vi "FiberMRI_Main.vi"() -> ()   [LabVIEW 2010]
doc: "Acquisition software for combined single-photon fluorescence and fMRI experiments."
uses:
  typedefs/acquisition_parameters_cluster.ctl
  typedefs/storage_parameters_cluster.ctl
  typedefs/experiment_mode_enum.ctl
  typedefs/stimulation_parameters.ctl
  typedefs/main_state_enum.ctl
  typedefs/control_daq_enum.ctl
  typedefs/control_display_enum.ctl
  typedefs/control_storage_enum.ctl
  typedefs/control_analysis_enum.ctl
  <vilib>/Utility/error.llb/DialogType.ctl
  typedefs/all_frontpanel_parameters.ctl
  <vilib>/ULx/Create Channel.llb/ULx Create Channel (DO-Digital Output).vi
  <vilib>/ULx/Write.llb/ULx Write (Digital Bool 1Line 1Point).vi
  globals/exit.vi
panel:
  out "Running":bool
  in  "Stimulation parameters":T1={"Physical channel"="Dev0/1stPortB/Do0", "Write chunk size"=1, "Sample rate"=1.0, "Stim onset"=0.0, "Stim frequency"=1.0, "ON time"=40.0, "OFF time"=120.0, "Repetitions"=1.0} {"Write chunk size" min=100 max=100000; "Sample rate" min=10.0 max=10000.0; "Repetitions" min=0.0 max=10.0 step=1.0; "OFF time" min=0.0 max=1000.0; "ON time" min=0.0 max=1000.0; "Stim onset" min=0.0 max=100.0; "Stim frequency" min=1.0 max=40.0 step=1.0}
  in  "Reset":bool
  in  "Shutter":bool
  in  "Experiment mode":T2
  in  "Storage parameters":T3
  in  "Acquisition parameters":T4={"Physical channels"="Dev0/Ai0:1", "Shutter line"="Dev0/1stPortA/Do0", "Clock source"=0, "Triggered?"=FALSE, "Sample rate"=1000.0, "Pixels to integrate"=1, "Effective data rate"=2000.0, "Read chunk size"=0, "Samples to read"=2000, "Run mode"=enum."Continuously"} {"Pixels to integrate" min=1 step=1; "Sample rate" min=10.0 max=25000.0; "Clock source" items=["OnboardClock", "ExternalClock", "NoClock"]}
  in  "Run":bool
  in  "Quit":bool
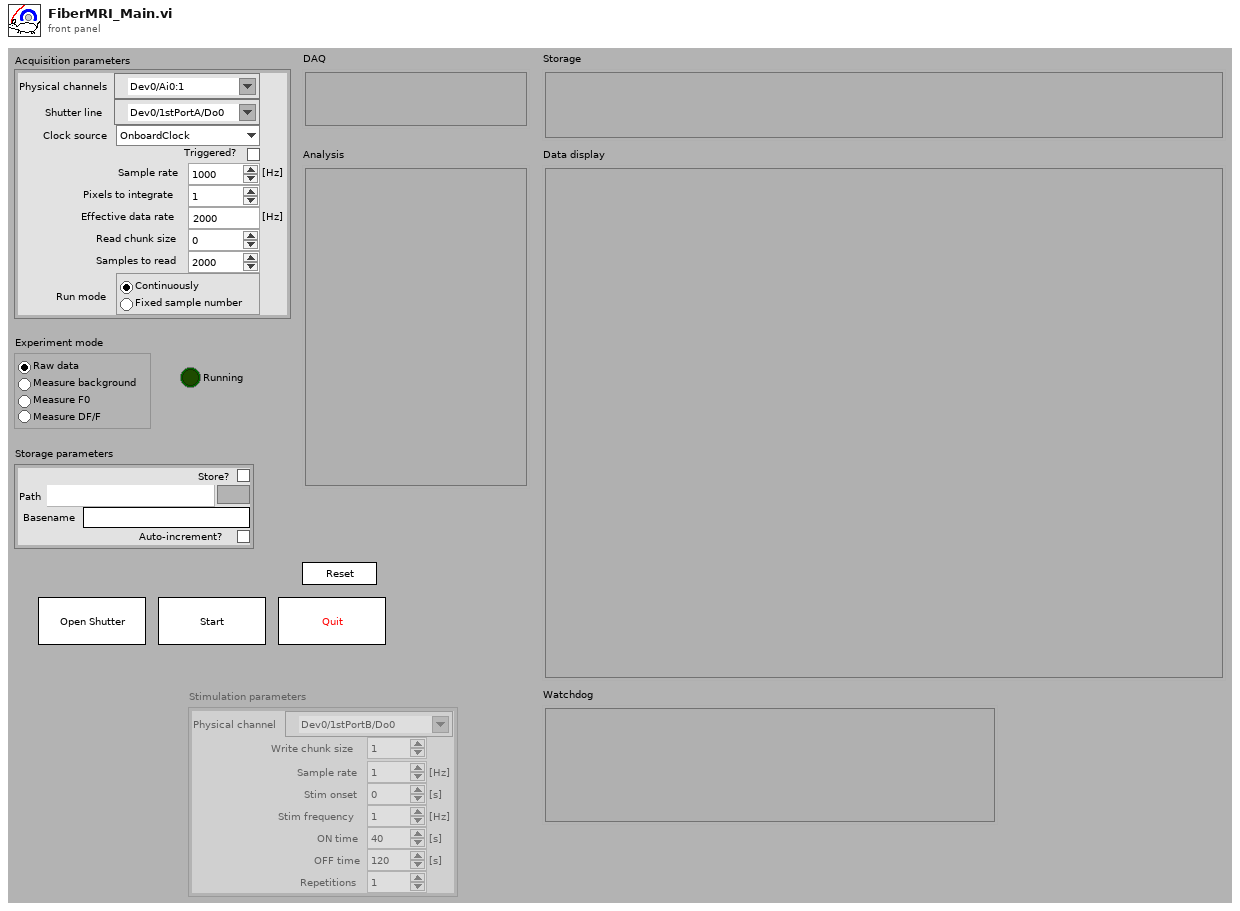
[diagram p1: front panel]
types:
  T1 = typedef "stimulation_parameters.ctl" = cluster{"Physical channel":tag, "Write chunk size":i32, "Sample rate":dbl, "Stim onset":dbl, "Stim frequency":dbl, "ON time":dbl, "OFF time":dbl, "Repetitions":dbl}
  T2 = typedef "experiment_mode_enum.ctl" = enum32{"Raw data", "Measure background", "Measure F0", "Measure DF/F"}
  T3 = typedef "storage_parameters_cluster.ctl" = cluster{"Store?":bool, "Path":path, "Basename":string, "Auto-increment?":bool}
  T4 = typedef "acquisition_parameters_cluster.ctl" = cluster{"Physical channels":refnum<k21>, "Shutter line":refnum<k21>, "Clock source":i32, "Triggered?":bool, "Sample rate":dbl, "Pixels to integrate":i32, "Effective data rate":dbl, "Read chunk size":i32, "Samples to read":i32, "Run mode":enum32{"Continuously", "Fixed sample number"}}
  T5 = typedef "all_frontpanel_parameters.ctl" = cluster{"Acquisition parameters":T4, "Experiment mode":T2, "Storage parameters":T3, "Stimulation parameters":T1}
  T6 = typedef "DialogType.ctl" = u16
  T7 = typedef "main_state_enum.ctl" = enum16{"Init", "ParamsChanged", "Start", "Stop", "SetShutter", "Reset", "Save", "Quit"}
  T8 = cluster{"Control_DAQ_Queue":refnum<queue>, "Control_Storage_Queue":refnum<queue>, "Control_Display_Queue":refnum<queue>, "Control_Analysis_Queue":refnum<queue>}
  T9 = typedef "control_analysis_enum.ctl" = enum16{"Init", "Analyze", "Reset", "Stop", "Quit"}
  T10 = cluster{"Control Analysis Enum":T9, "variant":variant}
  T11 = typedef "control_display_enum.ctl" = enum16{"Init", "Display", "Quit"}
  T12 = cluster{"Control display enum":T11, "variant":variant}
  T13 = typedef "control_storage_enum.ctl" = enum16{"Init", "Discard", "Store", "Reset", "Stop", "Quit"}
  T14 = cluster{"Control storage enum":T13, "variant":variant}
  T15 = typedef "control_daq_enum.ctl" = enum16{"Init", "GetCont", "GetNoSamples", "Stop", "Quit"}
  T16 = cluster{"Control DAQ Enum":T15, "variant":variant}
  T17 = cluster{"Acquisition parameters":T4, "Stimulation parameters":T1}
  T18 = cluster{"Control DAQ Enum":T15, "Variant":variant}
  T19 = cluster{"Experiment mode":T2, "Pixels to integrate":i32, "#channels":i32, "Iteration":i32}
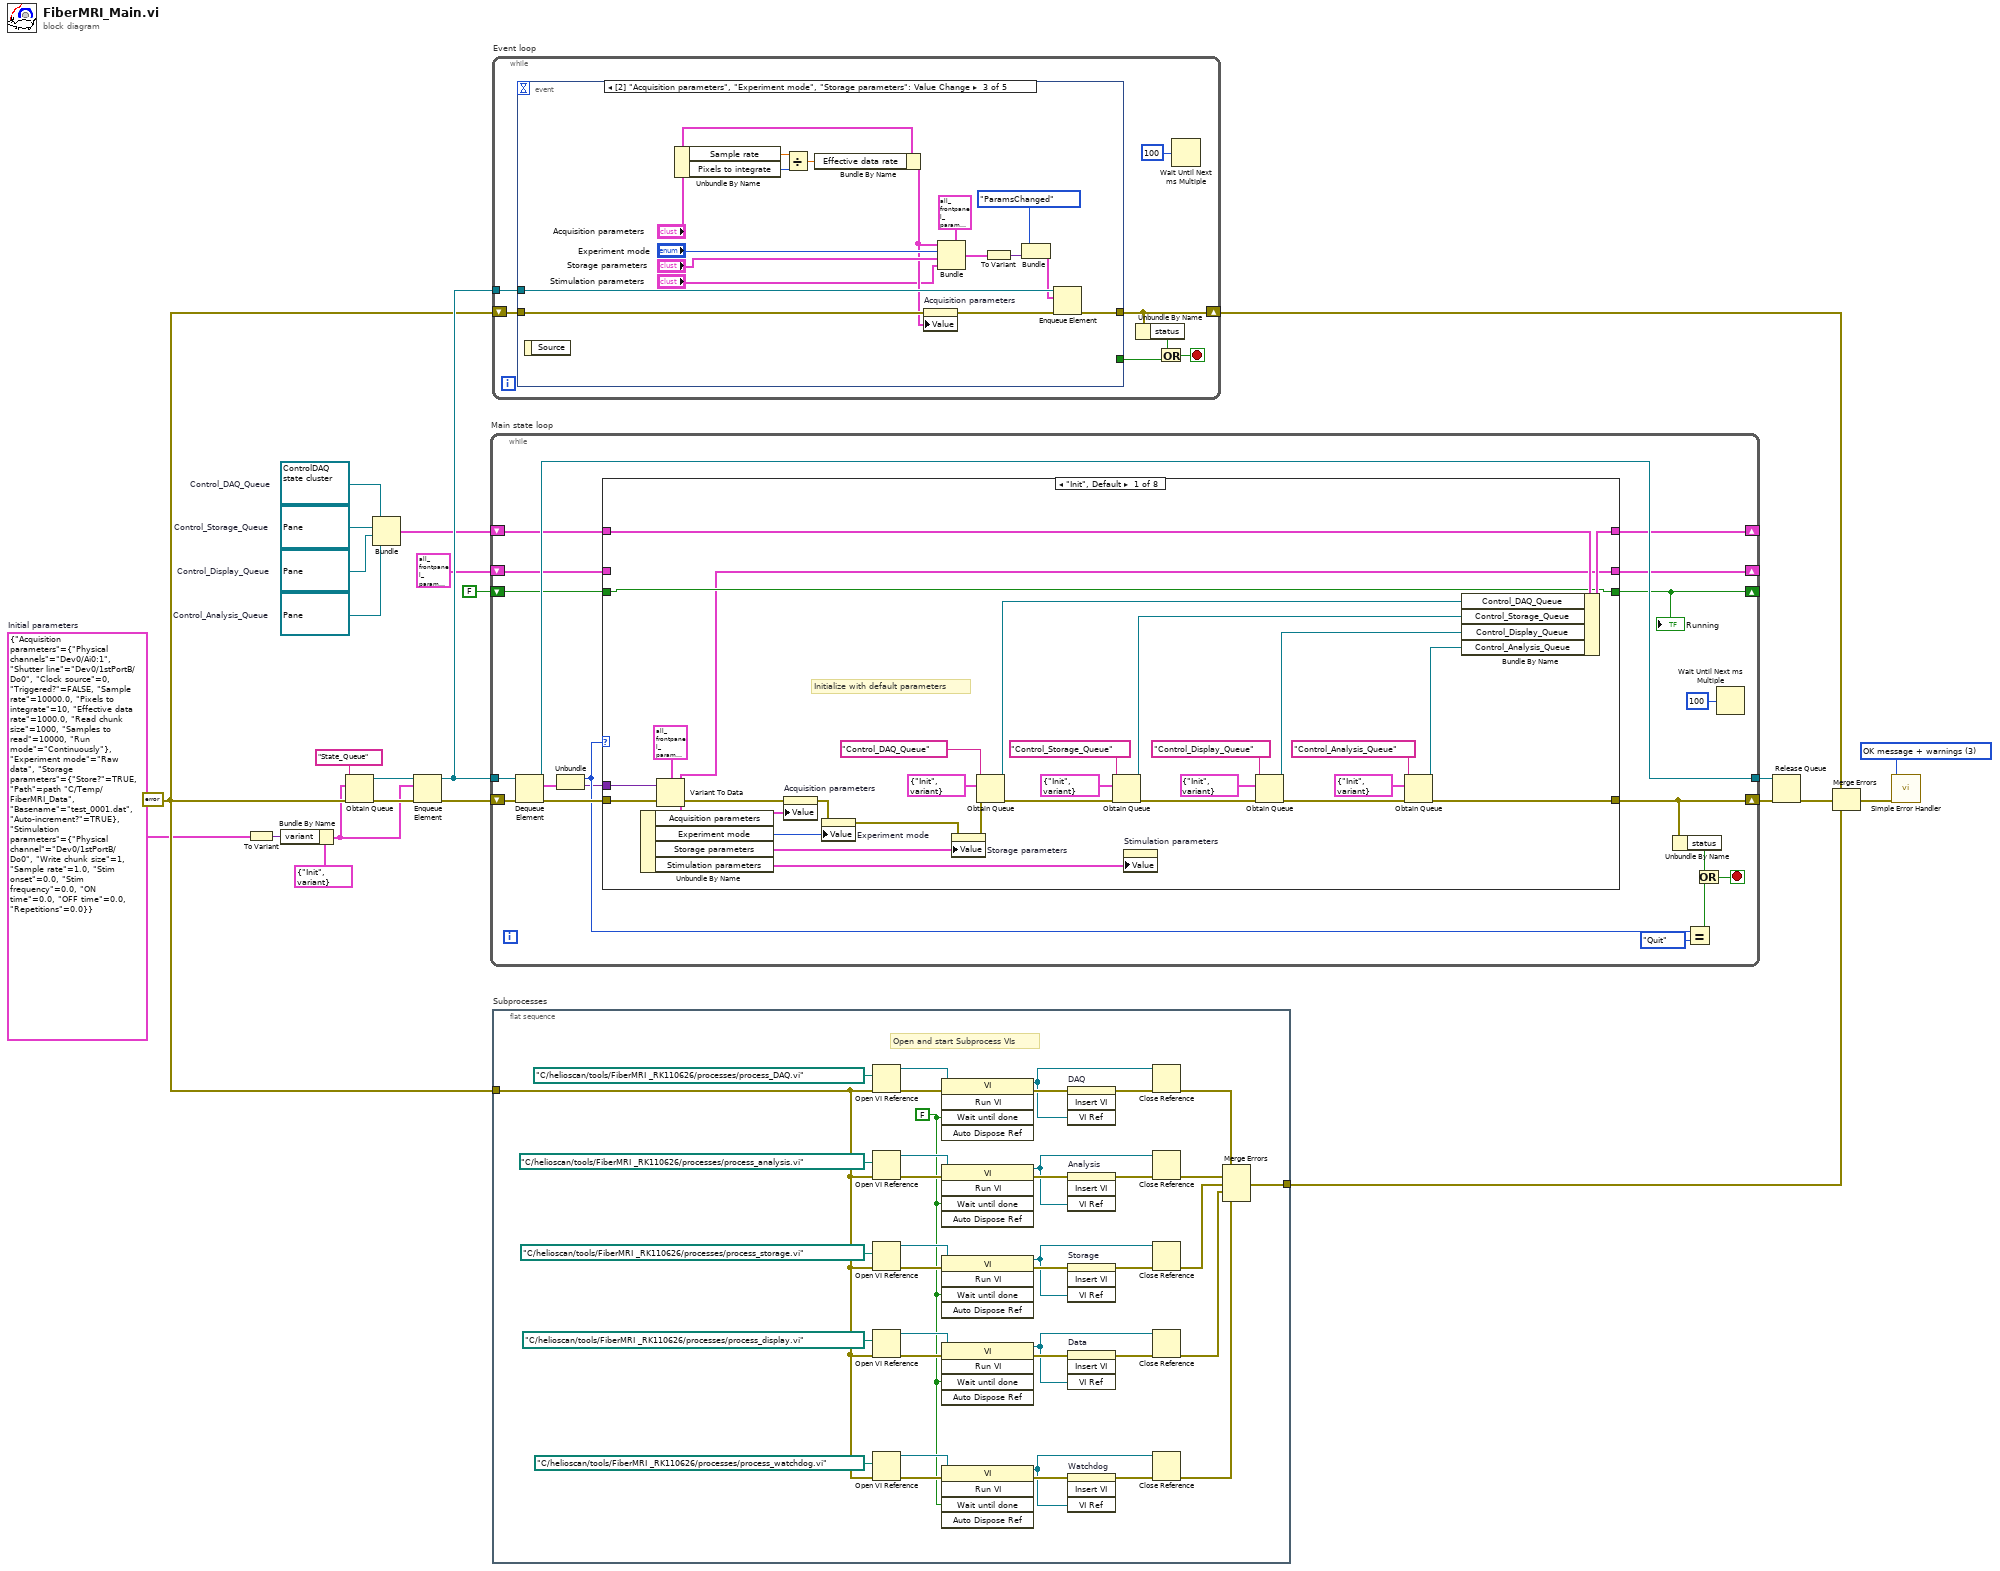
[diagram p0: block diagram]
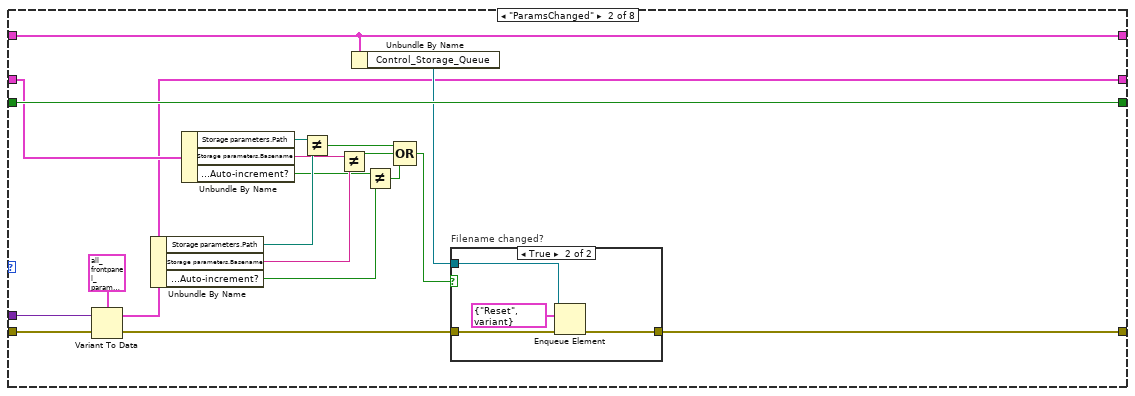
[diagram p2: hidden frame]
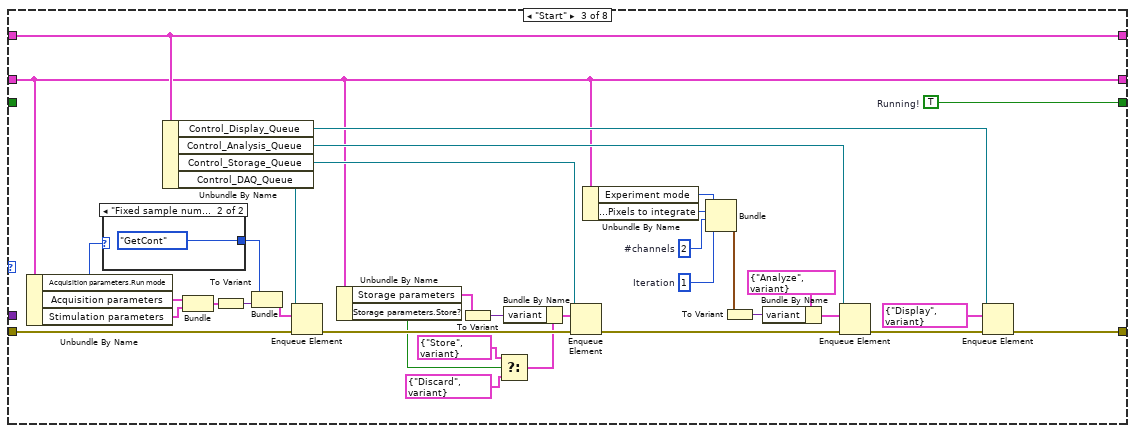
[diagram p4: hidden frame]
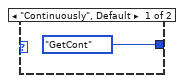
[diagram p5: hidden frame]
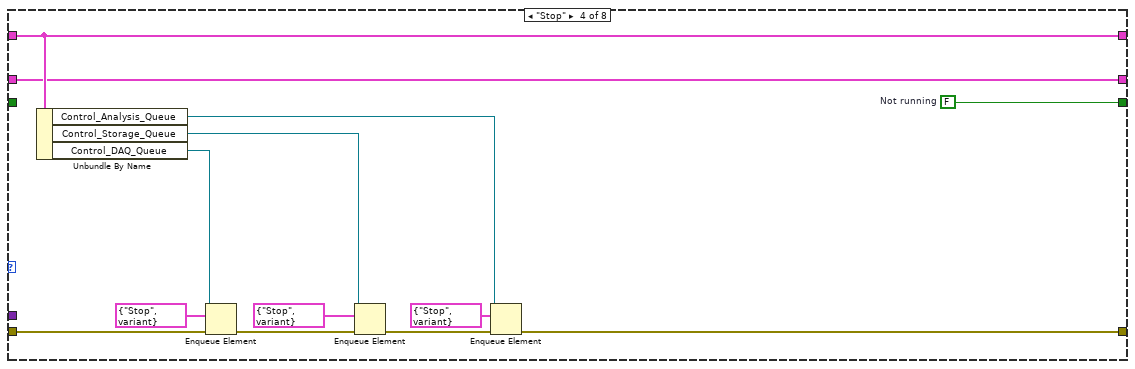
[diagram p6: hidden frame]
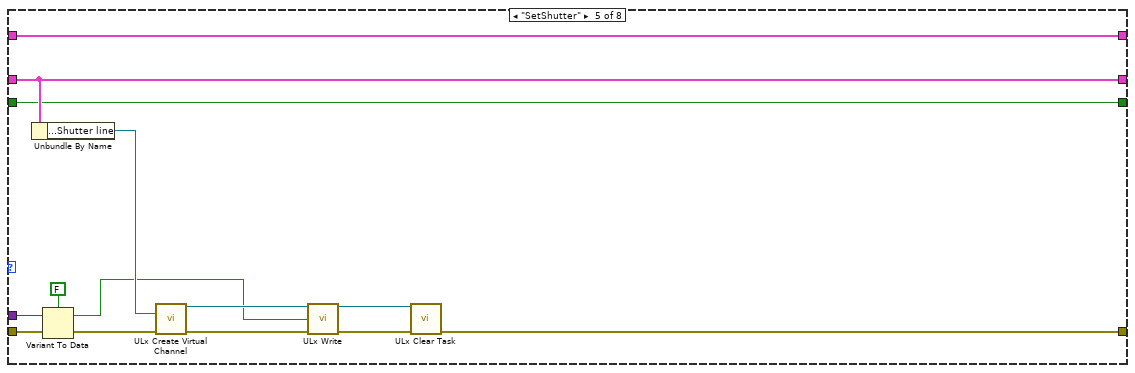
[diagram p7: hidden frame]
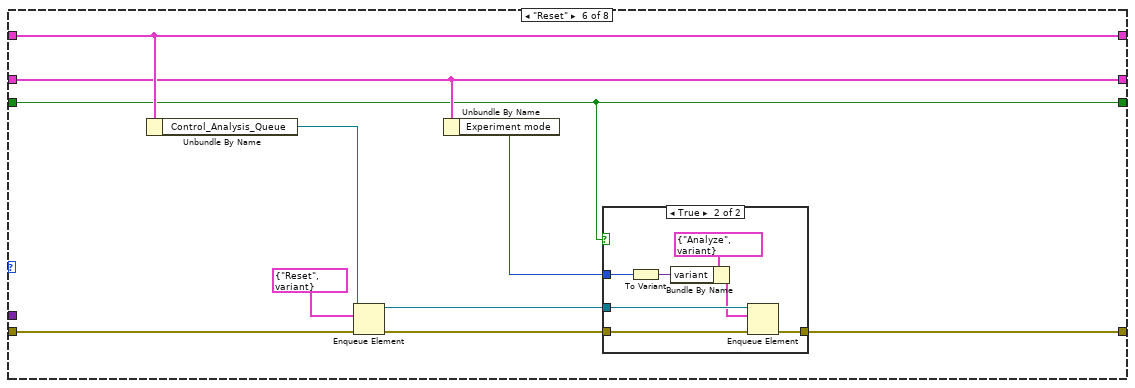
[diagram p8: hidden frame]
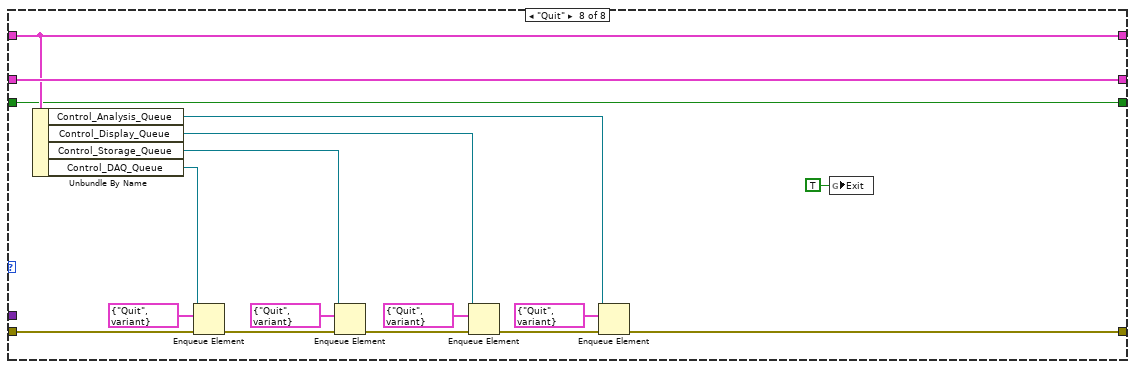
[diagram p11: hidden frame]
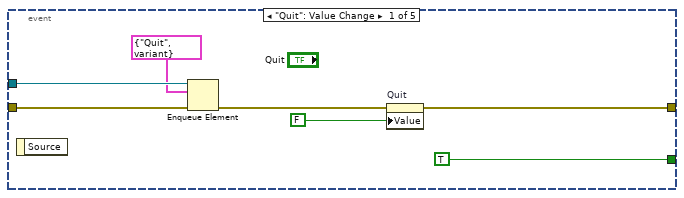
[diagram p12: hidden frame]
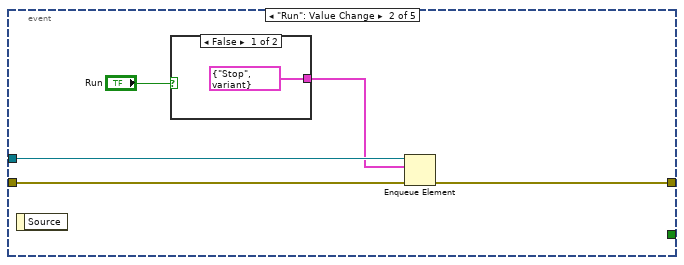
[diagram p13: hidden frame]
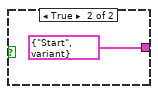
[diagram p14: hidden frame]
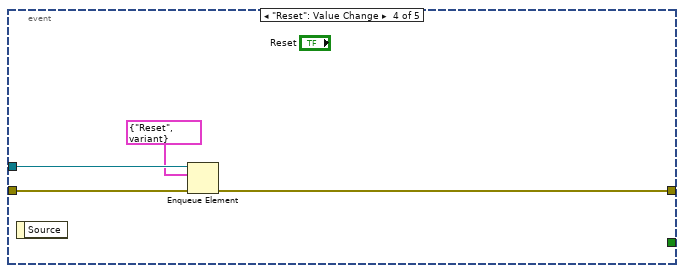
[diagram p15: hidden frame]
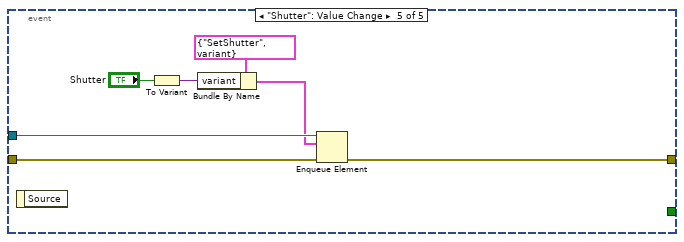
[diagram p16: hidden frame]
diagram:
  w1 = T5 {"Acquisition parameters"={"Physical channels"="Dev0/Ai0:1", "Shutter line"="Dev0/1stPortB/Do0", "Clock source"=0, "Triggered?"=FALSE, "Sample rate"=10000.0, "Pixels to integrate"=10, "Effective data rate"=1000.0, "Read chunk size"=1000, "Samples to read"=10000, "Run mode"=enum."Continuously"}, "Experiment mode"=enum."Raw data", "Storage parameters"={"Store?"=TRUE, "Path"=path "C:/Temp/FiberMRI_Data", "Basename"="test_0001.dat", "Auto-increment?"=TRUE}, "Stimulation parameters"={"Physical channel"="Dev0/1stPortB/Do0", "Write chunk size"=1, "Sample rate"=1.0, "Stim onset"=0.0, "Stim frequency"=0.0, "ON time"=0.0, "OFF time"=0.0, "Repetitions"=0.0}}  # Initial parameters
  w12 = T6 3 items=["no dialog", "OK message", "continue or stop message", "OK message + warnings", "continue/stop + warnings"] ("type of dialog (OK msg:1)")
  w13 = refnum<queue> refnum  # Control_Analysis_Queue
  w14 = refnum<queue> refnum  # Control_Storage_Queue
  w15 = refnum<queue> refnum  # Control_Display_Queue
  w9 = errorcluster {"status"=FALSE, "code"=0, "source"=""} ("error out")
  w18 = refnum<queue> refnum  # Control_DAQ_Queue
  n1 = To Variant(anything=w1) -> (Variant=w3:variant)
  n2 = Bundle By Name(cluster=cluster{"State Enum":T7, "variant":variant} {"State Enum"=enum."Init", "variant"=variant}, "variant"=w3) -> (w2:cluster{"State Enum":T7, "variant":variant})
  n3 = Obtain Queue(name (unnamed)="State_Queue", element data type=w2, error in (no error)=w9) -> (queue out=w23:refnum<queue>, error out=w21:errorcluster)  [unwired: 2 in, 1 out]
  n4 = Bundle("Control_DAQ_Queue"=w18, "Control_Storage_Queue"=w14, "Control_Display_Queue"=w15, "Control_Analysis_Queue"=w13) -> (w17:T8)  [unwired: 1 in]
  n5 = Enqueue Element(queue=w23, element=w2, error in (no error)=w21) -> (queue out=w22:refnum<queue>, error out=w16:errorcluster)  [unwired: 1 in, 1 out]
  n6 = while "Main state loop" {
    shift-right: [w31] -> w24
    shift-left: w16 -> [w41]
    shift-right: [w35] -> _
    shift-left: T5 {"Acquisition parameters"={"Physical channels"="", "Shutter line"="", "Clock source"=0, "Triggered?"=FALSE, "Sample rate"=1000.0, "Pixels to integrate"=0, "Effective data rate"=0.0, "Read chunk size"=0, "Samples to read"=2000, "Run mode"=enum."Continuously"}, "Experiment mode"=enum."Raw data", "Storage parameters"={"Store?"=FALSE, "Path"=path "", "Basename"="", "Auto-increment?"=FALSE}, "Stimulation parameters"={"Physical channel"="Dev0/Ai0", "Write chunk size"=1, "Sample rate"=1.0, "Stim onset"=0.0, "Stim frequency"=0.0, "ON time"=0.0, "OFF time"=0.0, "Repetitions"=0.0}} ("All frontpanel parameters") -> [w34]
    tunnel: w22 -> [w43]
    tunnel: [w42] -> w20
    shift-right: [w32] -> _
    shift-left: w17 -> [w33]
    shift-right: [w26] -> _
    shift-left: FALSE -> [w27]
    stop <- w28 stop-if-true
    n7 = Dequeue Element(queue=w43, error in (no error)=w41) -> (queue out=w42:refnum<queue>, element=w38:cluster{"State Enum":T7, "variant":variant}, error out=w40:errorcluster)  [unwired: 1 in, 1 out]
    n8 = Unbundle(w38) -> ("State Enum"=w37:T7, "variant"=w36:variant)
    n9 = case shown="\"Init\", Default" w37 {
      tunnel: w40 -> [w49 w93 w134 w149 w158 w172 w185 w202]
      tunnel: [w44 w76 w125 w139 w151 w167 w185 w190] -> w31
      tunnel: w36 -> [w45 w94 _ _ w156 _ _ _]
      tunnel: [w46 w75 w115 w138 w162 w169 w184 w201] -> w35
      tunnel: w34 -> [_ w90 w115 w138 w162 w169 w184 w201]
      tunnel: w33 -> [w70 w79 w129 w147 w163 w173 w183 w199]
      tunnel: [w69 w79 w129 w147 w163 w173 w183 w199] -> w32
      tunnel: w27 -> [w57 w92 _ _ w150 w164 w182 w187]
      tunnel: [w57 w92 w116 w137 w150 w164 w182 w187] -> w26
      frame "Init", Default {
        # "Initialize with default parameters"
        n10 = Variant To Data(error in=w49, Variant=w45, type=T5 {"Acquisition parameters"={"Physical channels"="Dev0/Ai0:1", "Shutter line"="Dev0/1stPortA/Do0", "Clock source"=0, "Triggered?"=FALSE, "Sample rate"=10000.0, "Pixels to integrate"=10, "Effective data rate"=1000.0, "Read chunk size"=1000, "Samples to read"=10000, "Run mode"=enum."Continuously"}, "Experiment mode"=enum."Raw data", "Storage parameters"={"Store?"=FALSE, "Path"=path "", "Basename"="", "Auto-increment?"=FALSE}, "Stimulation parameters"={"Physical channel"="Dev0/1stPortB/Do0", "Write chunk size"=1, "Sample rate"=1.0, "Stim onset"=0.0, "Stim frequency"=0.0, "ON time"=0.0, "OFF time"=0.0, "Repetitions"=0.0}} ("All frontpanel parameters")) -> (error out=w48:errorcluster, data=w46:T5)
        n11 = Unbundle By Name(w46) -> ("Acquisition parameters"=w56:T4, "Experiment mode"=w55:T2, "Storage parameters"=w51:T3, "Stimulation parameters"=w50:T1)
        n12 = property on="Acquisition parameters" class="Clust (strict)"(error in=w48, "Value"=w56) -> (error out=w54:errorcluster)  [unwired: 1 in, 1 out]
        n13 = property on="Experiment mode" class="RadioBtnsControl (strict)"(error in=w54, "Value"=w55) -> (error out=w53:errorcluster)  [unwired: 1 in, 1 out]
        n14 = property on="Storage parameters" class="Clust (strict)"(error in=w53, "Value"=w51) -> (error out=w52:errorcluster)  [unwired: 1 in, 1 out]
        n15 = Obtain Queue(name (unnamed)="Control_DAQ_Queue", element data type=T16 {"Control DAQ Enum"=enum."Init", "variant"=variant} ("ControlDAQ state cluster"), error in (no error)=w52) -> (queue out=w68:refnum<queue>, error out=w66:errorcluster)  [unwired: 2 in, 1 out]
        n16 = Obtain Queue(name (unnamed)="Control_Storage_Queue", element data type=T14 {"Control storage enum"=enum."Init", "variant"=variant}, error in (no error)=w66) -> (queue out=w67:refnum<queue>, error out=w65:errorcluster)  [unwired: 2 in, 1 out]
        n17 = property on="Stimulation parameters" class="Clust (strict)"("Value"=w50) -> ()  [unwired: 2 in, 2 out]
        n18 = Obtain Queue(name (unnamed)="Control_Display_Queue", element data type=T12 {"Control display enum"=enum."Init", "variant"=variant}, error in (no error)=w65) -> (queue out=w62:refnum<queue>, error out=w61:errorcluster)  [unwired: 2 in, 1 out]
        n19 = Obtain Queue(name (unnamed)="Control_Analysis_Queue", element data type=T10 {"Control Analysis Enum"=enum."Init", "variant"=variant}, error in (no error)=w61) -> (queue out=w58:refnum<queue>, error out=w44:errorcluster)  [unwired: 2 in, 1 out]
        n20 = Bundle By Name(cluster=w70, "Control_DAQ_Queue"=w68, "Control_Storage_Queue"=w67, "Control_Display_Queue"=w62, "Control_Analysis_Queue"=w58) -> (w69:T8)
      }
      frame "ParamsChanged" {
        n21 = Variant To Data(error in=w93, Variant=w94, type=T5 {"Acquisition parameters"={"Physical channels"="", "Shutter line"="", "Clock source"=0, "Triggered?"=FALSE, "Sample rate"=1000.0, "Pixels to integrate"=0, "Effective data rate"=0.0, "Read chunk size"=0, "Samples to read"=2000, "Run mode"=enum."Continuously"}, "Experiment mode"=enum."Raw data", "Storage parameters"={"Store?"=FALSE, "Path"=path "", "Basename"="", "Auto-increment?"=FALSE}, "Stimulation parameters"={"Physical channel"="Dev0/Ai0", "Write chunk size"=1, "Sample rate"=1.0, "Stim onset"=0.0, "Stim frequency"=0.0, "ON time"=0.0, "OFF time"=0.0, "Repetitions"=0.0}} ("All frontpanel parameters")) -> (error out=w77:errorcluster, data=w75:T5)
        n22 = Unbundle By Name(w75) -> ("Storage parameters.Path"=w88:path, "Storage parameters.Basename"=w86:string, "Storage parameters.Auto-increment?"=w84:bool)
        n23 = Unbundle By Name(w90) -> ("Storage parameters.Path"=w89:path, "Storage parameters.Basename"=w87:string, "Storage parameters.Auto-increment?"=w85:bool)
        n24 = Not Equal?(x=w89, y=w88) -> (x != y?=w83:bool)
        n25 = Not Equal?(x=w87, y=w86) -> (x != y?=w82:bool)
        n26 = Unbundle By Name(w79) -> ("Control_Storage_Queue"=w78:refnum<queue>)
        n27 = Not Equal?(x=w85, y=w84) -> (x != y?=w81:bool)
        n28 = Compound Arithmetic op=OR(w83, w82, w81) -> (w80:bool)
        n29 = case "Filename changed?" shown="True" w80 {
          tunnel: w78 -> [_ w99]
          tunnel: w77 -> [w95 w97]
          tunnel: [w95 w96] -> w76
          frame False {
          }
          frame True {
            n30 = Enqueue Element(queue=w99, element=T14 {"Control storage enum"=enum."Reset", "variant"=variant}, error in (no error)=w97) -> (error out=w96:errorcluster)  [unwired: 1 in, 2 out]
          }
        }
      }
      frame "Start" {
        w100 = 1  # Iteration
        w101 = 2  # #channels
        w116 = TRUE  # Running!
        n31 = Unbundle By Name(w115) -> ("Acquisition parameters.Run mode"=w131:enum32{"Continuously", "Fixed sample number"}, "Acquisition parameters"=w110:T4, "Stimulation parameters"=w109:T1)
        n32 = case shown="\"Fixed sample number\"" w131 {
          tunnel: [control_daq_enum."GetCont" ("Control DAQ Enum") control_daq_enum."GetCont" ("Control DAQ Enum")] -> w130
          frame "Continuously", Default {
          }
          frame "Fixed sample number" {
          }
        }
        n33 = Unbundle By Name(w129) -> ("Control_Display_Queue"=w123:refnum<queue>, "Control_Analysis_Queue"=w120:refnum<queue>, "Control_Storage_Queue"=w126:refnum<queue>, "Control_DAQ_Queue"=w128:refnum<queue>)
        n34 = Bundle("Acquisition parameters"=w110, "Stimulation parameters"=w109) -> (w108:T17)  [unwired: 1 in]
        n35 = To Variant(anything=w108) -> (Variant=w133:variant)
        n36 = Bundle("Control DAQ Enum"=w130, "Variant"=w133) -> (w132:T18)  [unwired: 1 in]
        n37 = Enqueue Element(queue=w128, element=w132, error in (no error)=w134) -> (error out=w127:errorcluster)  [unwired: 1 in, 2 out]
        n38 = Unbundle By Name(w115) -> ("Storage parameters"=w111:T3, "Storage parameters.Store?"=w106:bool)
        n39 = To Variant(anything=w111) -> (Variant=w107:variant)
        n40 = Select(t=T14 {"Control storage enum"=enum."Store", "variant"=variant} ("element"), s=w106, f=T14 {"Control storage enum"=enum."Discard", "variant"=variant} ("element")) -> (s? t:f=w103:T14)
        n41 = Bundle By Name(cluster=w103, "variant"=w107) -> (w102:T14)
        n42 = Enqueue Element(queue=w126, element=w102, error in (no error)=w127) -> (error out=w122:errorcluster)  [unwired: 1 in, 2 out]
        n43 = Unbundle By Name(w115) -> ("Experiment mode"=w114:T2, "Acquisition parameters.Pixels to integrate"=w113:i32)
        n44 = Bundle("Experiment mode"=w114, "Pixels to integrate"=w113, "#channels"=w101, "Iteration"=w100) -> (w112:T19)  [unwired: 1 in]
        n45 = To Variant(anything=w112) -> (Variant=w119:variant)
        n46 = Bundle By Name(cluster=T10 {"Control Analysis Enum"=enum."Analyze", "variant"=variant} ("element"), "variant"=w119) -> (w117:T10)
        n47 = Enqueue Element(queue=w120, element=w117, error in (no error)=w122) -> (error out=w121:errorcluster)  [unwired: 1 in, 2 out]
        n48 = Enqueue Element(queue=w123, element=T12 {"Control display enum"=enum."Display", "variant"=variant}, error in (no error)=w121) -> (error out=w125:errorcluster)  [unwired: 1 in, 2 out]
      }
      frame "Stop" {
        w137 = FALSE  # Not running
        n49 = Unbundle By Name(w147) -> ("Control_Analysis_Queue"=w141:refnum<queue>, "Control_Storage_Queue"=w144:refnum<queue>, "Control_DAQ_Queue"=w146:refnum<queue>)
        n50 = Enqueue Element(queue=w146, element=T16 {"Control DAQ Enum"=enum."Stop", "variant"=variant}, error in (no error)=w149) -> (error out=w145:errorcluster)  [unwired: 1 in, 2 out]
        n51 = Enqueue Element(queue=w144, element=T14 {"Control storage enum"=enum."Stop", "variant"=variant}, error in (no error)=w145) -> (error out=w142:errorcluster)  [unwired: 1 in, 2 out]
        n52 = Enqueue Element(queue=w141, element=T10 {"Control Analysis Enum"=enum."Stop", "variant"=variant}, error in (no error)=w142) -> (error out=w139:errorcluster)  [unwired: 1 in, 2 out]
      }
      frame "SetShutter" {
        n53 = Unbundle By Name(w162) -> ("Acquisition parameters.Shutter line"=w161:refnum<k21>)
        n54 = Variant To Data(error in=w158, Variant=w156, type=FALSE) -> (error out=w157:errorcluster, data=w154:bool)
        n55 = call-poly <vilib>:"ULx Create Virtual Channel.vi"("lines"=w161, "error in"=w157) -> ("task out"=w159:refnum<k24>, "error out"=w160:errorcluster)  [unwired: 12 in]
        n56 = call-poly <vilib>:"ULx Write.vi"("task in"=w159, "data"=w154, "error in"=w160) -> ("task out"=w153:refnum<k24>, "error out"=w152:errorcluster)  [unwired: 10 in, 1 out]
        n57 = call <vilib>:"ULx Clear Task.vi"("task in"=w153, "error in"=w152) -> ("error out"=w151:errorcluster)  [unwired: 13 in]
      }
      frame "Reset" {
        n58 = Unbundle By Name(w173) -> ("Control_Analysis_Queue"=w171:refnum<queue>)
        n59 = Enqueue Element(queue=w171, element=T10 {"Control Analysis Enum"=enum."Reset", "variant"=variant}, error in (no error)=w172) -> (queue out=w166:refnum<queue>, error out=w168:errorcluster)  [unwired: 1 in, 1 out]
        n60 = Unbundle By Name(w169) -> ("Experiment mode"=w165:T2)
        n61 = case shown="True" w164 {
          tunnel: [w174 w180] -> w167
          tunnel: w168 -> [w174 w181]
          tunnel: w166 -> [_ w179]
          tunnel: w165 -> [_ w178]
          frame False {
          }
          frame True {
            n62 = To Variant(anything=w178) -> (Variant=w175:variant)
            n63 = Bundle By Name(cluster=T10 {"Control Analysis Enum"=enum."Analyze", "variant"=variant} ("element"), "variant"=w175) -> (w176:T10)
            n64 = Enqueue Element(queue=w179, element=w176, error in (no error)=w181) -> (error out=w180:errorcluster)  [unwired: 1 in, 2 out]
          }
        }
      }
      frame "Save" {
      }
      frame "Quit" {
        n65 = Unbundle By Name(w199) -> ("Control_Analysis_Queue"=w189:refnum<queue>, "Control_Display_Queue"=w193:refnum<queue>, "Control_Storage_Queue"=w196:refnum<queue>, "Control_DAQ_Queue"=w198:refnum<queue>)
        n66 = Enqueue Element(queue=w198, element=T16 {"Control DAQ Enum"=enum."Quit", "variant"=variant} ("ControlDAQ state cluster"), error in (no error)=w202) -> (error out=w197:errorcluster)  [unwired: 1 in, 2 out]
        n67 = Enqueue Element(queue=w196, element=T14 {"Control storage enum"=enum."Quit", "variant"=variant}, error in (no error)=w197) -> (error out=w194:errorcluster)  [unwired: 1 in, 2 out]
        n68 = Enqueue Element(queue=w193, element=T12 {"Control display enum"=enum."Quit", "variant"=variant}, error in (no error)=w194) -> (error out=w191:errorcluster)  [unwired: 1 in, 2 out]
        n69 = Enqueue Element(queue=w189, element=T10 {"Control Analysis Enum"=enum."Quit", "variant"=variant}, error in (no error)=w191) -> (error out=w190:errorcluster)  [unwired: 1 in, 2 out]
        n70 = global write "exit.vi" "Exit"(TRUE ("Exit")) -> ()
      }
    }
    "Running" <- w26
    n71 = Unbundle By Name(w31) -> ("status"=w30:bool)
    n72 = Equal?(x=w37, y=main_state_enum."Quit") -> (x = y?=w29:bool)
    n73 = Or(x=w30, y=w29) -> (x .or. y?=w28:bool)
    n74 = Wait Until Next ms Multiple(millisecond multiple=u32 100) -> ()  [unwired: 1 out]
  }
  n75 = while "Event loop" {
    shift-right: [w205] -> w10
    shift-left: w9 -> [w208]
    tunnel: w22 -> [w209]
    stop <- w206 stop-if-true
    n76 = event shown="[2] \"Acquisition parameters\", \"Experiment mode\", \"Storage parameters\": Value Change" {
      selector: _ -> [_ _ _ _ _]
      dyn-events: _ -> [_ _ _ _ _]
      timeout: _ -> [_ _ _ _ _]
      tunnel: w209 -> [w215 w220 w240 w243 w250]
      tunnel: w208 -> [w216 w219 w227 w244 w251]
      tunnel: [w211 w217 w229 w242 w245] -> w205
      tunnel: [TRUE _ _ _ _] -> w207
      event "Quit": Value Change {
        n77 = event-data() -> ()  [unwired: 1 in, 1 out]
        n78 = Enqueue Element(queue=w215, element=cluster{"State Enum":T7, "variant":variant} {"State Enum"=enum."Quit", "variant"=variant}, error in (no error)=w216) -> (error out=w212:errorcluster)  [unwired: 1 in, 2 out]
        n79 = property on="Quit" class="Bool (strict)"(error in=w212, "Value"=FALSE) -> (error out=w211:errorcluster)  [unwired: 1 in, 1 out]
      }
      event "Run": Value Change {
        n80 = event-data() -> ()  [unwired: 1 in, 1 out]
        n81 = case shown="False" "Run" {
          tunnel: [cluster{"State Enum":T7, "variant":variant} {"State Enum"=enum."Stop", "variant"=variant} cluster{"State Enum":T7, "variant":variant} {"State Enum"=enum."Start", "variant"=variant}] -> w218
          frame False {
          }
          frame True {
          }
        }
        n82 = Enqueue Element(queue=w220, element=w218, error in (no error)=w219) -> (error out=w217:errorcluster)  [unwired: 1 in, 2 out]
      }
      event Value Change {
        n83 = event-data() -> ()  [unwired: 1 in, 1 out]
        n84 = Unbundle By Name("Acquisition parameters") -> ("Sample rate"=w232:dbl, "Pixels to integrate"=w233:i32)
        n85 = Divide(x=w232, y=w233) -> (x/y=w230:dbl)
        n86 = Bundle By Name(cluster="Acquisition parameters", "Effective data rate"=w230) -> (w226:T4)
        n87 = property on="Acquisition parameters" class="Clust (strict)"(error in=w227, "Value"=w226) -> (error out=w228:errorcluster)  [unwired: 1 in, 1 out]
        n88 = Bundle(cluster=T5 {"Acquisition parameters"={"Physical channels"="", "Shutter line"="", "Clock source"=0, "Triggered?"=FALSE, "Sample rate"=1000.0, "Pixels to integrate"=0, "Effective data rate"=0.0, "Read chunk size"=0, "Samples to read"=2000, "Run mode"=enum."Continuously"}, "Experiment mode"=enum."Raw data", "Storage parameters"={"Store?"=FALSE, "Path"=path "", "Basename"="", "Auto-increment?"=FALSE}, "Stimulation parameters"={"Physical channel"="Dev0/Ai0", "Write chunk size"=1, "Sample rate"=1.0, "Stim onset"=0.0, "Stim frequency"=0.0, "ON time"=0.0, "OFF time"=0.0, "Repetitions"=0.0}} ("All frontpanel parameters"), "Acquisition parameters"=w226, "Experiment mode"="Experiment mode", "Storage parameters"="Storage parameters", "Stimulation parameters"="Stimulation parameters") -> (w235:T5)
        n89 = To Variant(anything=w235) -> (Variant=w239:variant)
        n90 = Bundle("State Enum"=main_state_enum."ParamsChanged", "Variant"=w239) -> (w237:cluster{"State Enum":T7, "Variant":variant})  [unwired: 1 in]
        n91 = Enqueue Element(queue=w240, element=w237, error in (no error)=w228) -> (error out=w229:errorcluster)  [unwired: 1 in, 2 out]
      }
      event "Reset": Value Change {
        n92 = event-data() -> ()  [unwired: 1 in, 1 out]
        n93 = Enqueue Element(queue=w243, element=cluster{"State Enum":T7, "variant":variant} {"State Enum"=enum."Reset", "variant"=variant}, error in (no error)=w244) -> (error out=w242:errorcluster)  [unwired: 1 in, 2 out]
      }
      event "Shutter": Value Change {
        n94 = event-data() -> ()  [unwired: 1 in, 1 out]
        n95 = To Variant(anything="Shutter") -> (Variant=w248:variant)
        n96 = Bundle By Name(cluster=cluster{"State Enum":T7, "variant":variant} {"State Enum"=enum."SetShutter", "variant"=variant} ("element"), "variant"=w248) -> (w246:cluster{"State Enum":T7, "variant":variant})
        n97 = Enqueue Element(queue=w250, element=w246, error in (no error)=w251) -> (error out=w245:errorcluster)  [unwired: 1 in, 2 out]
      }
    }
    n98 = Unbundle By Name(w205) -> ("status"=w204:bool)
    n99 = Or(x=w204, y=w207) -> (x .or. y?=w206:bool)
    n100 = Wait Until Next ms Multiple(millisecond multiple=u32 100) -> ()  [unwired: 1 out]
  }
  n101 = flat-sequence "Subprocesses" {
    tunnel: w9 -> [w267]
    tunnel: [w269] -> w6
    frame #0 {
      w260 = FALSE ("Wait Until Done")
      # "Open and start Subprocess VIs"
      n102 = Open VI Reference(vi path=path "C:/helioscan/tools/FiberMRI _RK110626/processes/process_DAQ.vi", error in (no error)=w267) -> (vi reference=w284:refnum<vi>, error out=w285:errorcluster)  [unwired: 4 in]
      n103 = Open VI Reference(vi path=path "C:/helioscan/tools/FiberMRI _RK110626/processes/process_analysis.vi", error in (no error)=w267) -> (vi reference=w282:refnum<vi>, error out=w283:errorcluster)  [unwired: 4 in]
      n104 = Open VI Reference(vi path=path "C:/helioscan/tools/FiberMRI _RK110626/processes/process_storage.vi", error in (no error)=w267) -> (vi reference=w280:refnum<vi>, error out=w281:errorcluster)  [unwired: 4 in]
      n105 = Open VI Reference(vi path=path "C:/helioscan/tools/FiberMRI _RK110626/processes/process_display.vi", error in (no error)=w267) -> (vi reference=w278:refnum<vi>, error out=w279:errorcluster)  [unwired: 4 in]
      n106 = Open VI Reference(vi path=path "C:/helioscan/tools/FiberMRI _RK110626/processes/process_watchdog.vi", error in (no error)=w267) -> (vi reference=w265:refnum<vi>, error out=w268:errorcluster)  [unwired: 4 in]
      n107 = invoke class="VI" method="Run VI"(reference=w284, error in=w285, "Wait until done"=w260) -> (reference out=w257:refnum<vi>, error out=w259:errorcluster)  [unwired: 2 in, 3 out]
      n108 = invoke class="VI" method="Run VI"(reference=w282, error in=w283, "Wait until done"=w260) -> (reference out=w274:refnum<vi>, error out=w277:errorcluster)  [unwired: 2 in, 3 out]
      n109 = invoke class="VI" method="Run VI"(reference=w280, error in=w281, "Wait until done"=w260) -> (reference out=w252:refnum<vi>, error out=w255:errorcluster)  [unwired: 2 in, 3 out]
      n110 = invoke class="VI" method="Run VI"(reference=w278, error in=w279, "Wait until done"=w260) -> (reference out=w272:refnum<vi>, error out=w276:errorcluster)  [unwired: 2 in, 3 out]
      n111 = invoke class="VI" method="Run VI"(reference=w265, error in=w268, "Wait until done"=w260) -> (reference out=w262:refnum<vi>, error out=w264:errorcluster)  [unwired: 2 in, 3 out]
      n112 = invoke on="DAQ" class="SubPanel" method="Insert VI"(error in=w259, "VI Ref"=w257) -> (error out=w258:errorcluster)  [unwired: 2 in, 3 out]
      n113 = invoke on="Analysis" class="SubPanel" method="Insert VI"(error in=w277, "VI Ref"=w274) -> (error out=w275:errorcluster)  [unwired: 2 in, 3 out]
      n114 = invoke on="Storage" class="SubPanel" method="Insert VI"(error in=w255, "VI Ref"=w252) -> (error out=w254:errorcluster)  [unwired: 2 in, 3 out]
      n115 = invoke on="Data" class="SubPanel" method="Insert VI"(error in=w276, "VI Ref"=w272) -> (error out=w273:errorcluster)  [unwired: 2 in, 3 out]
      n116 = invoke on="Watchdog" class="SubPanel" method="Insert VI"(error in=w264, "VI Ref"=w262) -> (error out=w263:errorcluster)  [unwired: 2 in, 3 out]
      n117 = Close Reference(reference=w257, error in (no error)=w258) -> (error out=w256:errorcluster)
      n118 = Close Reference(reference=w274, error in (no error)=w275) -> (error out=w270:errorcluster)
      n119 = Close Reference(reference=w252, error in (no error)=w254) -> (error out=w253:errorcluster)
      n120 = Close Reference(reference=w272, error in (no error)=w273) -> (error out=w271:errorcluster)
      n121 = Close Reference(reference=w262, error in (no error)=w263) -> (error out=w261:errorcluster)
      n122 = Merge Errors(w256, w270, w253, w271, w261) -> (w269:errorcluster)
    }
  }
  n123 = Release Queue(queue=w20, error in (no error)=w24) -> (error out=w8:errorcluster)  [unwired: 1 in, 2 out]
  n124 = Merge Errors(w10, w8, w6) -> (w11:errorcluster)
  n125 = call <vilib>:"Simple Error Handler.vi"("type of dialog (OK msg:1)"=w12, "error in (no error)"=w11) -> ()  [unwired: 3 in, 5 out]
